vi "Sequence.CreateLocalVariables.vi"(8 "error in (no error)":errorcluster, 10 "Steps":T1[](array[typedef]), 11 "Sequence Ref":refnum<k24>) -> (0 "error out":errorcluster, 3 "Sequence Ref out":refnum<k24>)   [LabVIEW 2013, in "Simple Sequence Tools - Editor.lvlib"]
uses:
  Simple Sequence Tools - Editor.lvlib
  NationalInstruments.VeriStand.RealTimeSequenceDefinitionApi
  Types/Compiled.StepProperties.ctl
  Types/Compiled.IOStateProperties.ctl
  Types/Compiled.StepElementProperties.ctl
  Shared/Types/Channel.Properties.ctl
  Shared/Types/Step.Types.ctl
  Types/Compiled.StepCondition.ctl
  Types/Conditions.OperationTypes.ctl
  Shared/SubVIs/Main.Constants.vi
  Shared/Simple Sequence Tools - Shared.lvlib
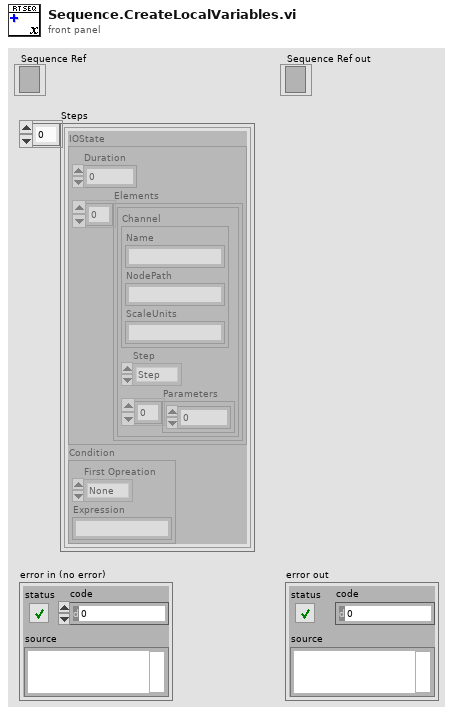
[diagram p1: front panel]
types:
  T1 = typedef "Simple Sequence Tools - Editor.lvlib/Compiled.StepProperties.ctl" = cluster{"IOState":T2, "Condition":T6}
  T2 = typedef "Simple Sequence Tools - Editor.lvlib/Compiled.IOStateProperties.ctl" = cluster{"Duration":dbl, "Elements":T3[]}
  T3 = typedef "Simple Sequence Tools - Editor.lvlib/Compiled.StepElementProperties.ctl" = cluster{"Channel":T4, "Step":T5, "Parameters":dbl[]}
  T4 = typedef "Simple Sequence Tools - Shared.lvlib/Channel.Properties.ctl" = cluster{"Name":string, "NodePath":string, "ScaleUnits":string}
  T5 = typedef "Simple Sequence Tools - Shared.lvlib/Step.Types.ctl" = enum8{"Step", "iStep", "Ramp", "Unchanged", "Unknown", "Sine", "SweptSine"}
  T6 = typedef "Simple Sequence Tools - Editor.lvlib/Compiled.StepCondition.ctl" = cluster{"First Opreation":T7, "Expression":string}
  T7 = typedef "Simple Sequence Tools - Editor.lvlib/Conditions.OperationTypes.ctl" = enum8{"None", "&&", "||"}
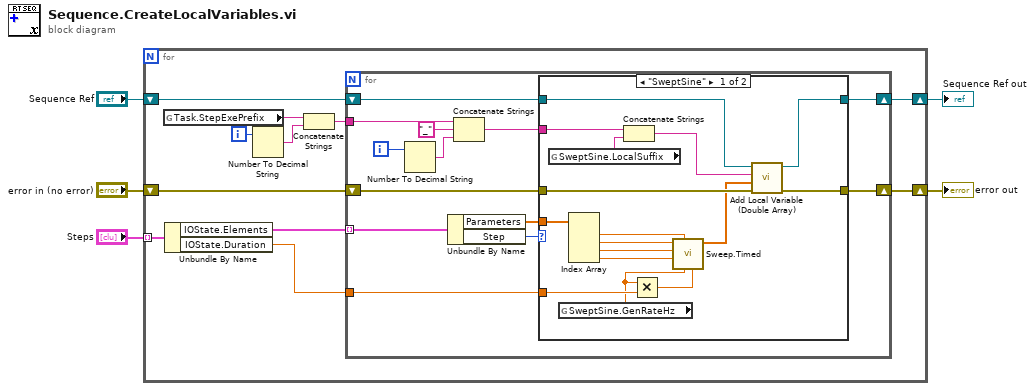
[diagram p0: block diagram]
diagram:
  n1 = for {
    tunnel: "Steps" -> [w16] mode=indexing
    shift-right: [w11] -> w3
    shift-left: "error in (no error)" -> [w12]
    shift-right: [w13] -> w5
    shift-left: "Sequence Ref" -> [w14]
    i -> [w10]
    n2 = global read "Main.Constants.vi" "Task.StepExePrefix"() -> (w9:string)
    n3 = Unbundle By Name(w16) -> ("IOState.Elements"=w15:T3[], "IOState.Duration"=w6:dbl)
    n4 = Number To Decimal String(number=w10) -> (decimal integer string=w8:string)  [unwired: 1 in]
    n5 = Concatenate Strings(w9, w8) -> (w7:string)
    n6 = for {
      tunnel: w15 -> [w29] mode=indexing
      shift-right: [w23] -> w13
      shift-left: w14 -> [w24]
      shift-right: [w22] -> w11
      shift-left: w12 -> [w28]
      tunnel: w6 -> [w26]
      tunnel: w7 -> [w18]
      i -> [w19]
      n7 = Number To Decimal String(number=w19) -> (decimal integer string=w21:string)  [unwired: 1 in]
      n8 = Unbundle By Name(w29) -> ("Parameters"=w27:dbl[], "Step"=w25:T5)
      n9 = Concatenate Strings(w18, "_" ("string"), w21) -> (w17:string)
      n10 = case shown="\"SweptSine\"" w25 {
        tunnel: w28 -> [w43 w46]
        tunnel: w27 -> [w45 _]
        tunnel: w26 -> [w44 _]
        tunnel: w24 -> [w42 w47]
        tunnel: [w41 w47] -> w23
        tunnel: [w40 w46] -> w22
        tunnel: w17 -> [w37 _]
        frame "SweptSine" {
          n11 = global read "Main.Constants.vi" "SweptSine.LocalSuffix"() -> (w36:string)
          n12 = global read "Main.Constants.vi" "SweptSine.GenRateHz"() -> (w38:dbl)
          n13 = Index Array(array=w45) -> (element #1=w33:dbl, element #2=w34:dbl, element #3=w32:dbl, element #4=w31:dbl)  [unwired: 4 in]
          n14 = Concatenate Strings(w37, w36) -> (w35:string)
          n15 = Multiply(x=w38, y=w44) -> (x*y=w30:dbl)
          n16 = call "Sweep.Timed.vi"("DataPoints"=w30, "Fsample (S/s)"=w38, "Offset"=w33, "EndHz"=w31, "StartHz"=w32, "Amplitude"=w34) -> ("Chirp Data"=w39:dbl[])  [unwired: 4 in, 1 out]
          n17 = call "Add Local Variable (Double Array).vi"("error in (no error)"=w43, "Array"=w39, "Identifier"=w35, "Sequence Ref in"=w42) -> ("error out"=w40:errorcluster, "Sequence Ref out"=w41:refnum<k24>)  [unwired: 6 in]
        }
        frame Default {
        }
      }
    }
  }
  "Sequence Ref out" <- w5
  "error out" <- w3
